vi "Parse Pirani 2.vi"(11 "bytes in":string) -> (2 "DBL data":dbl, 3 "bytes out":string)   [LabVIEW 2019, in "PGC2D.lvlib"]
uses:
  PGC2D.lvlib
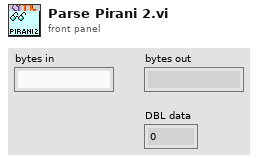
[diagram p1: front panel]
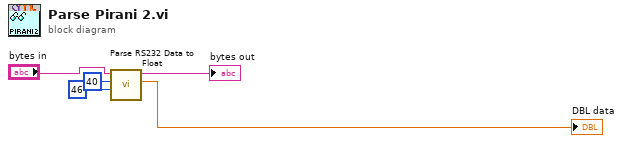
[diagram p0: block diagram]
diagram:
  n1 = call "Parse RS232 Data to Float.vi"("AML end byte"=46, "AML start byte"=40, "bytes in"="bytes in") -> ("DBL data"=→"DBL data":dbl, "bytes out"=→"bytes out":string)  [unwired: 7 in]
